vi "Configure Data Pattern.vi"(6 "Enable Differential Encoding (T:Enable)":bool=TRUE, 7 "4-Bit Repeating Sequence (0)":u16(ring) items=["0", "1", "2", "3", "4", "5", "6", "7", "8", "9", "10", "11", "12", "13", "14", "15"], 8 "error in (no error)":errorcluster, 9 "File Name (\"\")":string, 10 "Data Pattern (4: PN23)":u16(ring)=4 items=["PN9", "PN11", "PN15", "PN20", "PN23", "FIX4", "Select File", "External", "4 1's & 4 0's", "8 1's & 8 0's", "16 1's & 16 0's", "32 1's & 32 0's", "64 1's & 64 0's", "PRAM File"], 11 "VISA resource name":refnum<visa-resource-name>) -> (0 "error out":errorcluster, 3 "VISA resource name out":refnum<visa-resource-name>)   [LabVIEW 2012, in "Agilent PSG MXG Series.lvlib"]
doc: "Configures data pattern for unframed transmission.\n\n<B>Notes:</B>\n(1) This VI is valid only in E8267C, E8267D, N5172B, N5182B.\n\n(2) For E8267C, this VI is valid only when the instrument installs <B>Option 002</B> (Internal baseband generator) or <B>Option 602</B> (Digital bus baseband generator).\n\n(3) For E8267D, this VI is valid only when the instrument installs <B>Option 601</B> or <B>Option 602</B> (Internal baseband generator).\n\n(4) For N5172B and N5182B, this VI is valid only when the instrument installs <B>Option 431</B>."
uses:
  <instrlib>/Agilent PSG MXG Series/Agilent PSG MXG Series.lvlib
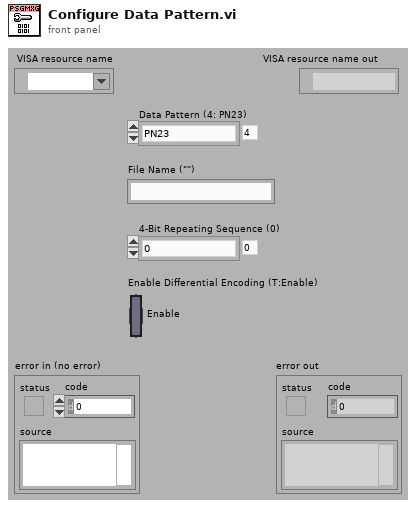
[diagram p1: front panel]
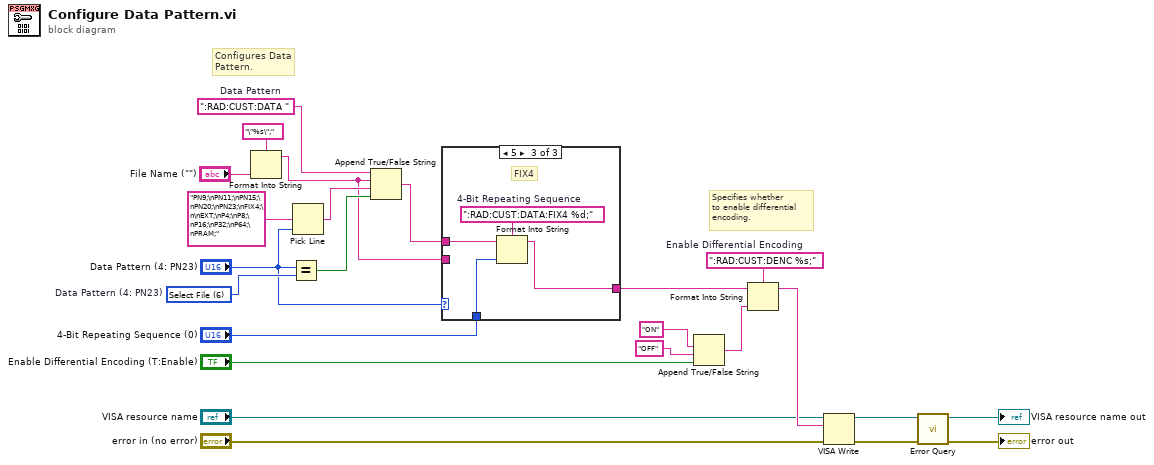
[diagram p0: block diagram]
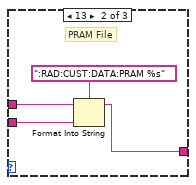
[diagram p3: hidden frame]
diagram:
  w10 = ":RAD:CUST:DENC %s;"  # Enable Differential Encoding
  w22 = ":RAD:CUST:DATA "  # Data Pattern
  w24 = u16 6 items=["PN9", "PN11", "PN15", "PN20", "PN23", "FIX4", "Select File", "External", "4 1's & 4 0's", "8 1's & 8 0's", "16 1's & 16 0's", "32 1's & 32 0's", "64 1's & 64 0's"]  # Data Pattern (4: PN23)
  # "Specifies whether\nto enable differential\nencoding."
  # "Configures Data\nPattern."
  n1 = Format Into String(format string="\"%s\";", "File Name (\"\")") -> (resulting string=w5:string)  [unwired: 2 in, 1 out]
  n2 = Equal?(x="Data Pattern (4: PN23)", y=w24) -> (x = y?=w23:bool)
  n3 = Pick Line(multi-line string="PN9;\nPN11;\nPN15;\nPN20;\nPN23;\nFIX4;\n\nEXT;\nP4;\nP8;\nP16;\nP32;\nP64;\nPRAM;", line index="Data Pattern (4: PN23)") -> (output string=w18:string)  [unwired: 1 out]
  n4 = Append True/False String(1:w23, 2:w18, 3:w5, 4:w22) -> (0:w17:string)
  n5 = case shown="5" "Data Pattern (4: PN23)" {
    tunnel: w17 -> [w25 w29 w33]
    tunnel: "4-Bit Repeating Sequence (0)" -> [_ _ w31]
    tunnel: [w25 w28 w30] -> w8
    tunnel: w5 -> [_ w26 _]
    frame 0, Default {
    }
    frame 13 {
      # "PRAM File"
      n6 = Format Into String(format string=":RAD:CUST:DATA:PRAM %s", initial string=w29, w26) -> (resulting string=w28:string)  [unwired: 1 in, 1 out]
    }
    frame 5 {
      w32 = ":RAD:CUST:DATA:FIX4 %d;"  # 4-Bit Repeating Sequence
      # "FIX4"
      n7 = Format Into String(format string=w32, initial string=w33, w31) -> (resulting string=w30:string)  [unwired: 1 in, 1 out]
    }
  }
  n8 = Append True/False String(1:"Enable Differential Encoding (T:Enable)", 2:"OFF" ("false string"), 3:"ON" ("true string")) -> (0:w7:string)  [unwired: 1 out]
  n9 = Format Into String(format string=w10, initial string=w8, w7) -> (resulting string=w6:string)  [unwired: 1 in, 1 out]
  n10 = VISA Write(VISA resource name="VISA resource name", write buffer=w6, error in (no error)="error in (no error)") -> (VISA resource name out=w12:refnum<visa-resource-name>, error out=w11:errorcluster)  [unwired: 1 out]
  n11 = call <instrlib>:"Error Query.vi"("error in (no error)"=w11, "VISA resource name"=w12) -> ("error out"=→"error out":errorcluster, "VISA resource name out"=→"VISA resource name out":refnum<visa-resource-name>)  [unwired: 8 out]
